vi "Greater than 0.vi"(11 "Rational Number in":refnum<class "Rational Number.lvclass">) -> (3 "Greater than 0?":bool)   [LabVIEW 2021, in "Rational Number.lvclass"]
uses:
  Rational Number.lvclass
  Rational Number.lvclass/Rational Number.ctl
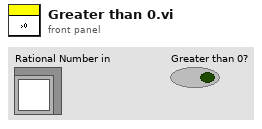
[diagram p1: front panel]
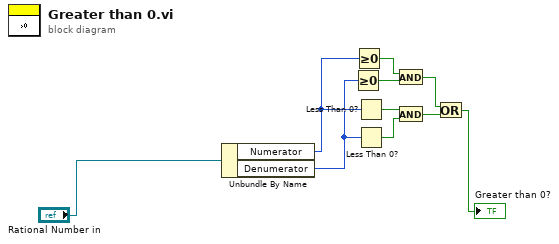
[diagram p0: block diagram]
diagram:
  n1 = Unbundle By Name("Rational Number in") -> ("Numerator"=w2:i64, "Denumerator"=w1:i64)
  n2 = Greater Or Equal To 0?(x=w1) -> (x >= 0?=w8:bool)
  n3 = Greater Or Equal To 0?(x=w2) -> (x >= 0?=w7:bool)
  n4 = Less Than 0?(x=w2) -> (x < 0?=w5:bool)
  n5 = Less Than 0?(x=w1) -> (x < 0?=w6:bool)
  n6 = And(x=w7, y=w8) -> (x .and. y?=w3:bool)
  n7 = And(x=w5, y=w6) -> (x .and. y?=w4:bool)
  n8 = Or(x=w3, y=w4) -> (x .or. y?=→"Greater than 0?":bool)
